vi "Where Am I (SubVI).vi"(0 "TL Calling Location":string, 1 "Call VI path":path) -> (2 "I'm here":string)   [LabVIEW 2015]
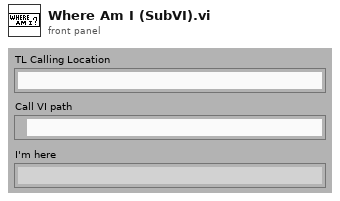
[diagram p1: front panel]
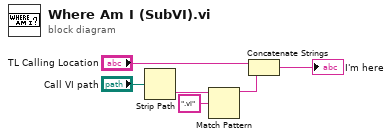
[diagram p0: block diagram]
diagram:
  n1 = Strip Path(path="Call VI path") -> (name=w3:string)  [unwired: 1 out]
  n2 = Match Pattern(string=w3, regular expression=".vi") -> (before substring=w5:string)  [unwired: 4 out]
  n3 = Concatenate Strings("TL Calling Location", w5) -> (→"I'm here":string)
